vi "HCC Get Viper Diagnostics.vi"(0 "GEA Ref In":refnum<k24>, 1 "GEA2 Event Registration":refnum<event-registration>, 2 "Diagnostic":T2, 3 "Input Data":T3 {"Command" format="%02x"; "Destination" format="%02x"; "Source" format="%02x"}, 5 "error in (no error)":errorcluster, 8 "Read Timeout (ms)":u32=5000) -> (14 "GEA Ref Out":refnum<k24>, 15 "Event Registration Out":refnum<event-registration>, 16 "Diagnostic Data Output":T2, 17 "Converted Data Out":T1 {"CRC" format="%04x"; "Length" format="%02x"; "Command" format="%02x"; "Destination" format="%02x"; "Source" format="%02x"}, 19 "error out":errorcluster)   [LabVIEW 2016]
uses:
  Type Definitions/ViperHawk/ViperHawk Diagnostic Data.ctl
  Utility/LabVIEW GEA2 Toolkit v1.0.0.0/type defs/Data In.ctl
  C:/Technology Lab/NI-2010/Trunk/Utility/LabVIEW GEA2 Toolkit v1.0.0.0/Appliance.NET/GeaCommunication.dll
  Utility/LabVIEW GEA2 Toolkit v1.0.0.0/Appliance.NET/GeaCommunication.dll
  Utility/LabVIEW GEA2 Toolkit v1.0.0.0/type defs/Data Out.ctl
  Utility/LabVIEW GEA2 Toolkit v1.0.0.0/library/GEA2_Toolkit.lvlib
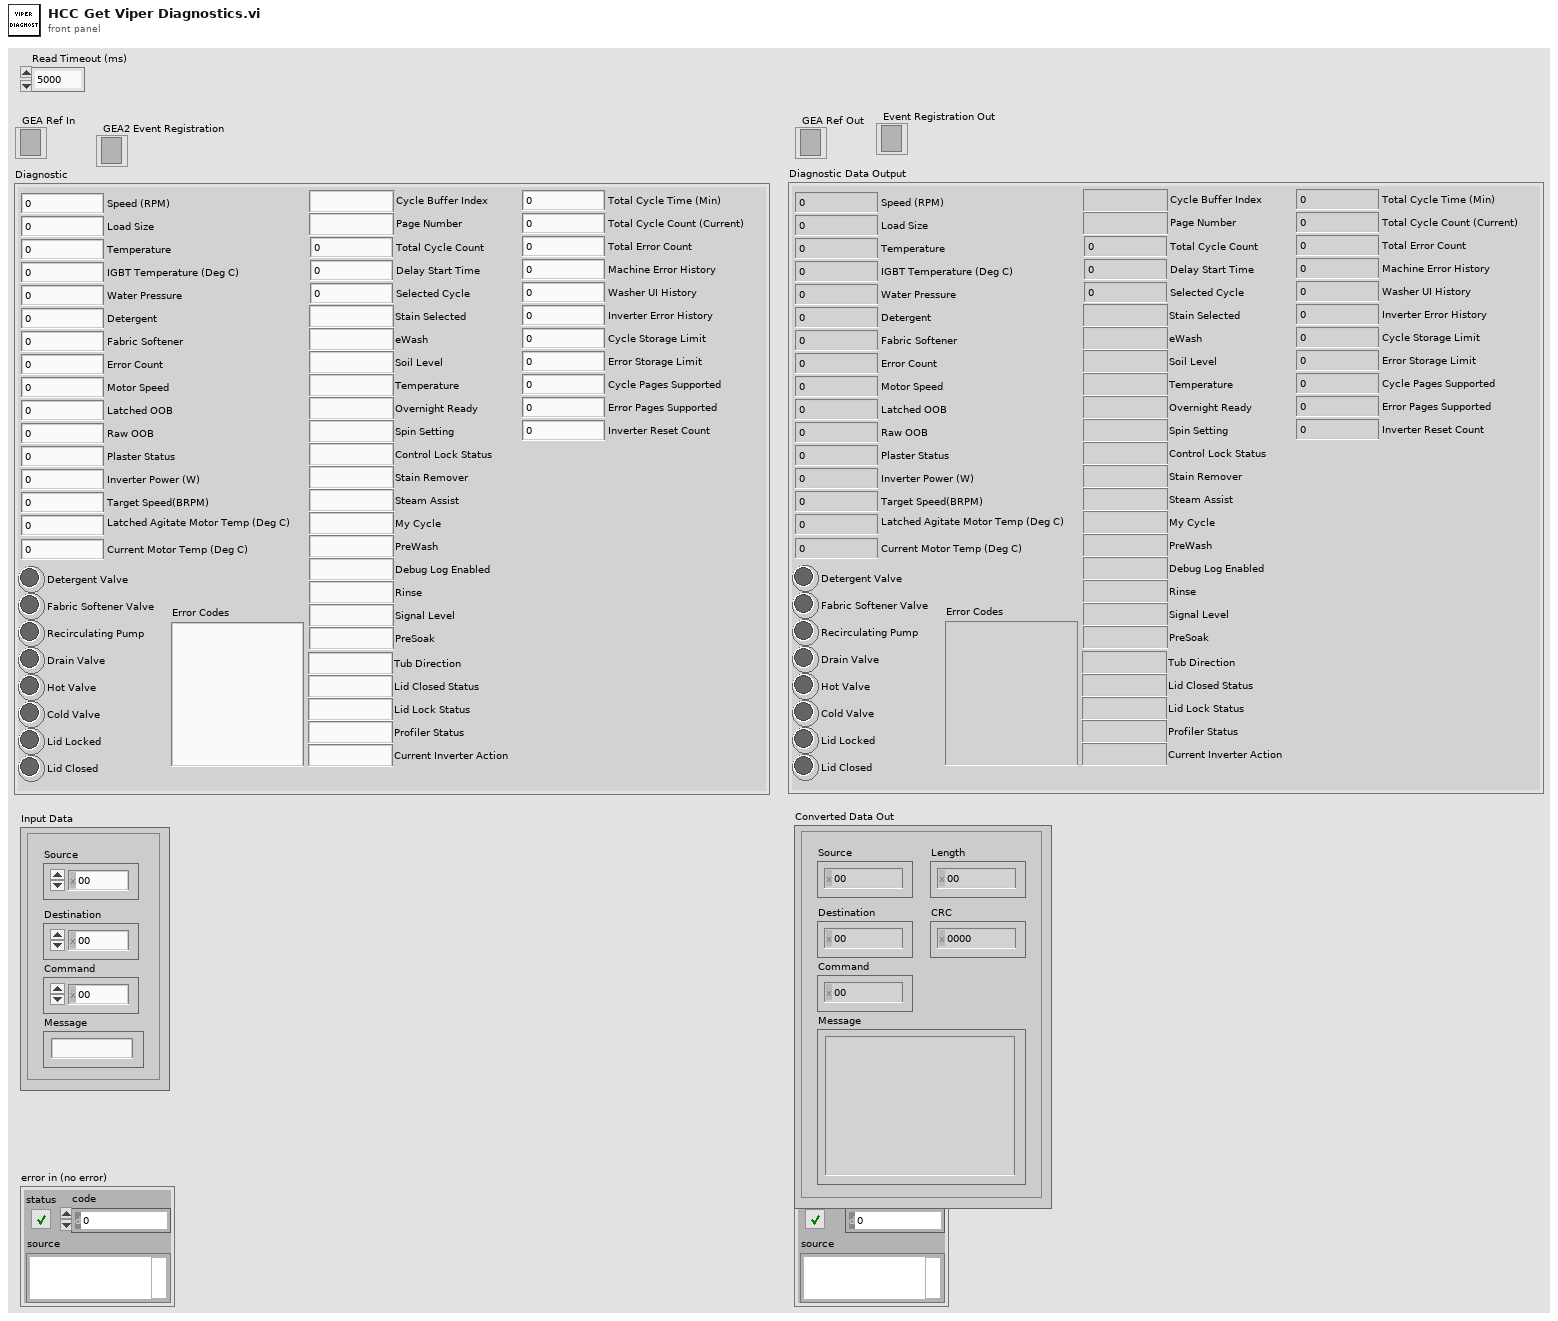
[diagram p1: front panel]
types:
  T1 = typedef "GEA2_Toolkit.lvlib/Data Out.ctl" = cluster{"Source":u8, "Destination":u8, "Command":u8, "Length":u8, "CRC":u16, "Message":string}
  T2 = typedef "ViperHawk Diagnostic Data.ctl" = cluster{"Speed (RPM)":u32, "Load Size":u32, "Temperature":u32, "Water Pressure":dbl, "Detergent":u32, "Fabric Softener":u32, "Tub Direction":string, "Detergent Valve":bool, "Fabric Softener Valve":bool, "Recirculating Pump":bool, "Drain Valve":bool, "Hot Valve":bool, "Cold Valve":bool, "Lid Closed Status":string, "Lid Lock Status":string, "Error Count":u32, "IGBT Temperature (Deg C)":u32, "Motor Speed":u32, "Latched OOB":u32, "Raw OOB":u32, "Plaster Status":u32, "Inverter Power (W)":u32, "Target Speed(BRPM)":u32, "Latched Agitate Motor Temp (Deg C)":u32, "Current Motor Temp (Deg C)":u32, "Profiler Status":string, "Current Inverter Action":string, "Error Codes":string, "Lid Locked":bool, "Lid Closed":bool, "9E Diagnostic Data":cluster{"Total Cycle Time (Min)":u32, "Total Cycle Count (Current)":u16, "Total Error Count":u16, "Machine Error History":u32, "Washer UI History":u32, "Inverter Error History":u32, "Cycle Storage Limit":u8, "Error Storage Limit":u8, "Cycle Pages Supported":u8, "Error Pages Supported":u8, "Inverter Reset Count":u16}, "9F Diagnostic Data":cluster{"Cycle Buffer Index":string, "Page Number":string, "Total Cycle Count":u32, "Delay Start Time":u32, "Stain Selected":string, "Selected Cycle":u32, "eWash":string, "Soil Level":string, "Temperature":string, "Overnight Ready":string, "Spin Setting":string, "Control Lock Status":string, "Stain Remover":string, "Steam Assist":string, "My Cycle":string, "PreWash":string, "Debug Log Enabled":string, "Rinse":string, "Signal Level":string, "PreSoak":string}}
  T3 = typedef "GEA2_Toolkit.lvlib/Data In.ctl" = cluster{"Source":u8, "Destination":u8, "Command":u8, "Message":string}
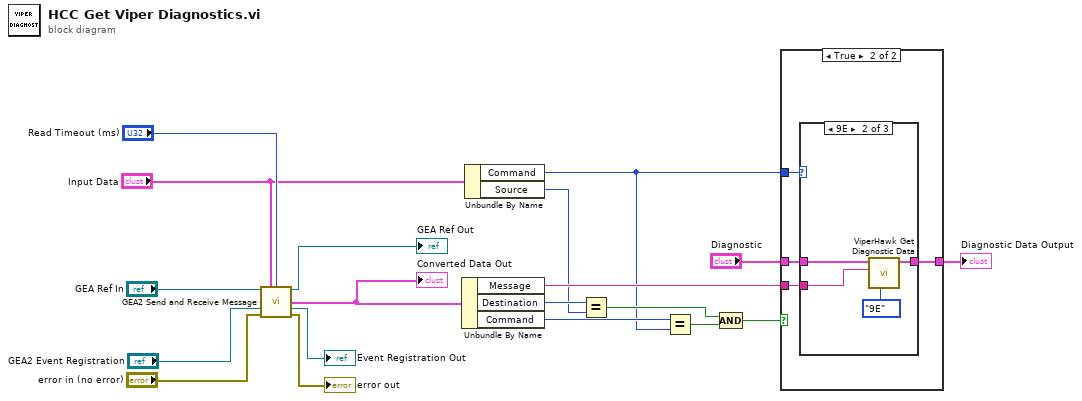
[diagram p0: block diagram]
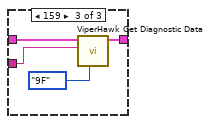
[diagram p4: hidden frame]
diagram:
  n1 = call "GEA2 Send and Receive Message.vi"("GEA2 Reference In"="GEA Ref In", "Input Data"="Input Data", "Read Timeout (ms)"="Read Timeout (ms)", "GEA2 Event Registration"="GEA2 Event Registration", "Error In"="error in (no error)") -> ("GEA2 Reference Out"=→"GEA Ref Out":refnum<k24>, "Converted Data Out"=w12:T1, "Event Registration Out"=→"Event Registration Out":refnum<event-registration>, "Error Out"=→"error out":errorcluster)  [unwired: 5 in, 2 out]
  "Converted Data Out" <- w12
  n2 = Unbundle By Name(w12) -> ("Message"=w7:string, "Destination"=w6:u8, "Command"=w8:u8)
  n3 = Unbundle By Name("Input Data") -> ("Command"=w2:u8, "Source"=w1:u8)
  n4 = Equal?(x=w6, y=w1) -> (x = y?=w9:bool)
  n5 = Equal?(x=w8, y=w2) -> (x = y?=w10:bool)
  n6 = Compound Arithmetic op=AND(w9, w10) -> (w11:bool)
  n7 = case shown="True" w11 {
    tunnel: w7 -> [_ w23]
    tunnel: "Diagnostic" -> [w20 w24]
    tunnel: [w20 w22] -> w19
    tunnel: w2 -> [_ w21]
    frame False {
    }
    frame True {
      n8 = case shown="9E" w21 {
        tunnel: w24 -> [w25 w29 w32]
        tunnel: w23 -> [_ w28 w31]
        tunnel: [w25 w27 w30] -> w22
        frame Default {
        }
        frame 158 {
          n9 = call "ViperHawk Get Diagnostic Data.vi"("Command"=enum16{"9E", "9F"}."9E", "Hex String In"=w28, "Diagnostic"=w29) -> ("Diagnostic Data Output"=w27:T2)  [unwired: 8 in]
        }
        frame 159 {
          n10 = call "ViperHawk Get Diagnostic Data.vi"("Command"=enum16{"9E", "9F"}."9F", "Hex String In"=w31, "Diagnostic"=w32) -> ("Diagnostic Data Output"=w30:T2)  [unwired: 8 in]
        }
      }
    }
  }
  "Diagnostic Data Output" <- w19
